vi "Inverse Kinematics.vi"   [LabVIEW 2017, in "NI_Kinematics.lvlib"]
doc: "Computes the joint angles of a robotic arm given the location of the end effector relative to the arm base. Wire data to the <B>end effector transform</B> input to determine the polymorphic instance to use or manually select the instance.\n\n<B>.m file:</B> ikine"
uses:
  <vilib>/robotics/Kinematics/NI_Kinematics.lvlib
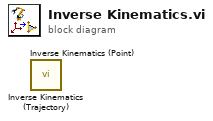
[diagram p0: block diagram]
diagram:
  n1 = call <vilib>:"Inverse Kinematics (Trajectory).vi"() -> ()  [unwired: 8 in, 4 out]
  n2 = call <vilib>:"Inverse Kinematics (Point).vi"() -> ()  [unwired: 8 in, 4 out]
